vi "set_and_meas_RMS_with_attenuator.vi"(7 "need_attenuator_notification":bool=TRUE caption="Уведомление об установке аттенюатора", 8 "error in (no error)":errorcluster, 9 "Frequency (Hz)":dbl, 10 "Amplitude (1.0 Vpp)":dbl, 11 "app_data in":T1) -> (0 "error out":errorcluster, 1 "boc_data":sgl[](array[numeric]), 2 "meas":dbl[](array[numeric]), 3 "output cluster out":T1)   [LabVIEW 2017]
uses:
  controls/attenuator_dB.ctl
  controls/app_data.ctl
  controls/instruments.ctl
  Unicorn Labview Library/Control/unicorn_Param.ctl
  Unicorn Labview Library/Control/unicorn_conn.ctl
  Unicorn Labview Library/Control/unicorn_JSON.ctl
  Unicorn Labview Library/Control/unicorn_ParamInt.ctl
  Unicorn Labview Library/Control/unicorn_Telemetry.ctl
  Unicorn Labview Library/Control/unicorn_Table.ctl
  Unicorn Labview Library/Control/unicorn_ParamFloat.ctl
  Unicorn Labview Library/Unicorn Library.lvlib
panel:
  out "Attenuator(dB)":T10
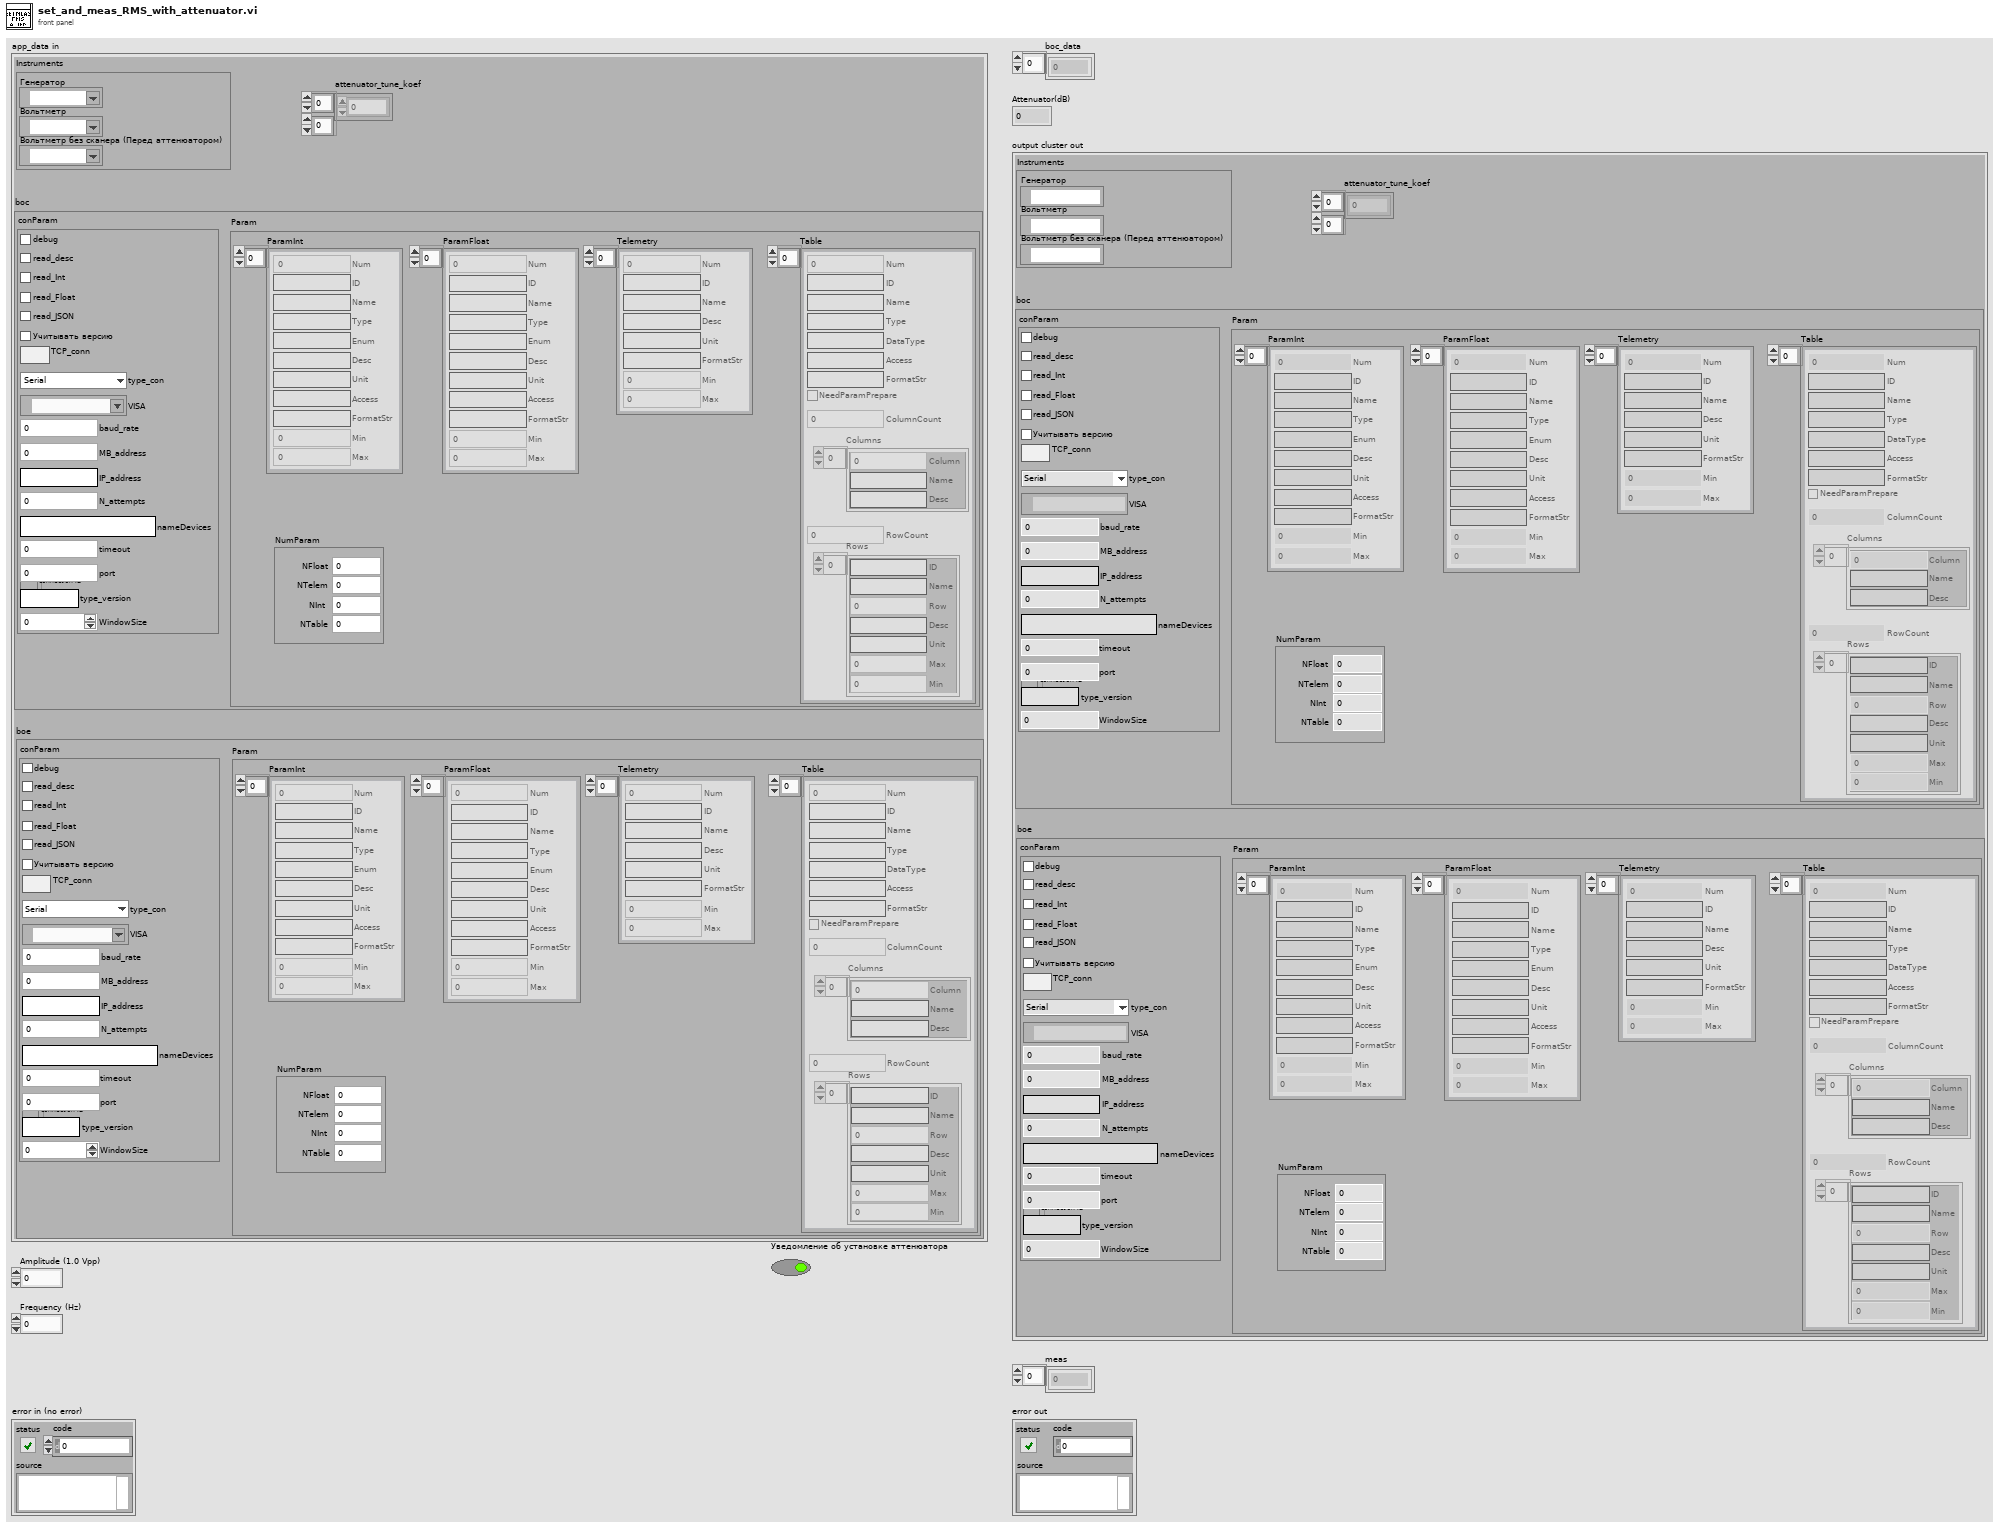
[diagram p1: front panel]
types:
  T1 = typedef "app_data.ctl" = cluster{"Instruments":T2, "boc":T3, "boe":T3, "attenuator_tune_koef":dbl[][]}
  T2 = typedef "instruments.ctl" = cluster{"generator":refnum<visa-resource-name>, "voltment_with_scaner":refnum<visa-resource-name>, "voltment_without_scaner":refnum<visa-resource-name>}
  T3 = typedef "Unicorn Library.lvlib/unicorn_Param.ctl" = cluster{"conParam":T4, "Param":T5}
  T4 = typedef "Unicorn Library.lvlib/unicorn_conn.ctl" = cluster{"ReadIntParam":bool, "ReadDescrParam":bool, "ReadFloatParam":bool, "debug":bool, "ReadJSON":bool, "IP_address":string, "N_attempts":i32, "type_con":enum16{"Serial", "TCP"}, "MB_address":i32, "VISA":refnum<visa-resource-name>, "connection ID":refnum<k5>, "nameDevices":string, "timeout":i32, "port":u16, "type_version":string, "baud_rate":u32, "VersionControl":bool, "TCP_conn":bool, "WindowSize":i32}
  T5 = typedef "Unicorn Library.lvlib/unicorn_JSON.ctl" = cluster{"NumParam":cluster{"NTelem":i32, "NInt":i32, "NFloat":i32, "NTable":i32}, "ParamInt":T6, "Telemetry":T7, "Table":T8, "ParamFloat":T9}
  T6 = typedef "Unicorn Library.lvlib/unicorn_ParamInt.ctl" = cluster{"ID":string, "Num":i32, "Name":string, "Type":string, "Enum":string, "Desc":string, "Unit":string, "Access":string, "FormatStr":string, "Min":i32, "Max":i32}[]
  T7 = typedef "Unicorn Library.lvlib/unicorn_Telemetry.ctl" = cluster{"ID":string, "Num":i32, "Name":string, "Desc":string, "Unit":string, "FormatStr":string, "Min":i32, "Max":i32}[]
  T8 = typedef "Unicorn Library.lvlib/unicorn_Table.ctl" = cluster{"Num":i32, "Access":string, "ColumnCount":i32, "NeedParamPrepare":bool, "Columns":cluster{"Column":i32, "Desc":string, "Name":string}[], "DataType":string, "FormatStr":string, "ID":string, "Name":string, "RowCount":i32, "Rows":cluster{"Desc":string, "ID":string, "Max":i32, "Min":i32, "Name":string, "Row":i32, "Unit":string}[], "Type":string}[]
  T9 = typedef "Unicorn Library.lvlib/unicorn_ParamFloat.ctl" = cluster{"ID":string, "Num":i32, "Name":string, "Type":string, "Enum":string, "Desc":string, "Unit":string, "Access":string, "FormatStr":string, "Min":i32, "Max":i32}[]
  T10 = typedef "attenuator_dB.ctl" = enum16{"0", "20", "40", "60"}
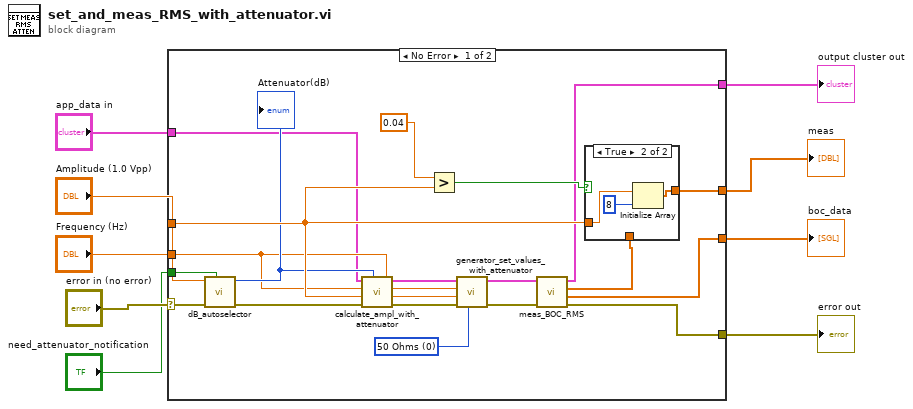
[diagram p0: block diagram]
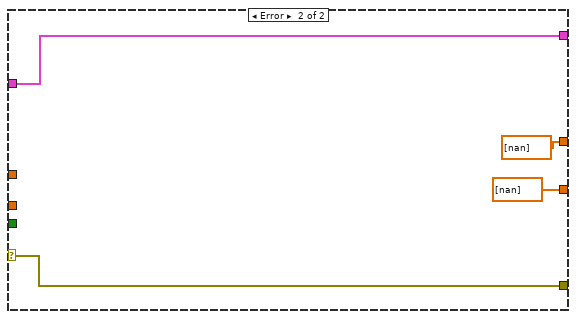
[diagram p3: hidden frame]
diagram:
  n1 = case shown="No Error" "error in (no error)" {
    selector: "error in (no error)" -> [w11 w37]
    tunnel: "Amplitude (1.0 Vpp)" -> [w28 _]
    tunnel: [w26 dbl[] [nan] ("meas")] -> w8
    tunnel: "Frequency (Hz)" -> [w22 _]
    tunnel: "app_data in" -> [w17 w36]
    tunnel: [w16 sgl[] [nan] ("boc_data")] -> w5
    tunnel: [w15 w37] -> w4
    tunnel: [w14 w36] -> w3
    tunnel: "need_attenuator_notification" -> [w10 _]
    frame No Error {
      w21 = u16 0 items=["50 Ohms", "High Impedance"] ("Impedance (0: 50 Ohms)")
      n2 = call "dB_autoselector.vi"("need_attenuator_notification"=w10, "error_in"=w11, "Amplitude"=w28) -> ("error_out"=w24:errorcluster, "Attenuator(dB)"=w23:T10)  [unwired: 7 in]
      "Attenuator(dB)" <- w23
      n3 = call "calculate_ampl_with_attenuator.vi"("Attenuator(dB)"=w23, "error in"=w24, "Amplitude_in"=w28, "frequency"=w22, "app_data in in"=w17) -> ("error out"=w18:errorcluster, "Amplitude_out"=w19:dbl, "app_data out"=w20:T1)  [unwired: 4 in]
      n4 = Greater?(x=0.04 ("y"), y=w28) -> (0:w29:bool)
      n5 = call "generator_set_values_with_attenuator.vi"("Impedance (0: 50 Ohms)"=w21, "error in (no error)"=w18, "Frequency (1000 Hz)"=w22, "Amplitude (1.0 Vpp)"=w19, "app_data"=w20) -> ("error out"=w13:errorcluster, "output cluster"=w12:T1)  [unwired: 5 in]
      n6 = call "meas_BOC_RMS.vi"("error in (no error)"=w13, "output cluster in"=w12) -> ("error out"=w15:errorcluster, "boc_data"=w16:sgl[], "meas"=w25:dbl[], "output cluster out"=w14:T1)  [unwired: 6 in]
      n7 = case shown="True" w29 {
        tunnel: w25 -> [w30 _]
        tunnel: [w30 w33] -> w26
        tunnel: w28 -> [_ w32]
        frame False {
        }
        frame True {
          n8 = Initialize Array(w32, 8 ("dimension size")) -> (w33:dbl[])
        }
      }
    }
    frame Error {
    }
  }
  "meas" <- w8
  "boc_data" <- w5
  "error out" <- w4
  "output cluster out" <- w3
